vi "Serial_ini.vi"(6 "error in":errorcluster, 7 "Serial path":path, 8 "Date":string, 9 "Count":i32, 10 "Shift":string, 11 "Enum":enum16{"Write", "Read"}(ring)) -> (0 "error out":errorcluster, 1 "Count":u32, 2 "Shift":string, 3 "Date":string)   [LabVIEW 2017]
uses:
  <vilib>/Utility/config.llb/Write Key (String).vi
  <vilib>/Utility/config.llb/Write Key (I32).vi
  <vilib>/Utility/config.llb/Read Key (String).vi
  <vilib>/Utility/config.llb/Read Key (U32).vi
  <vilib>/Utility/config.llb/NI_LVConfig.lvlib
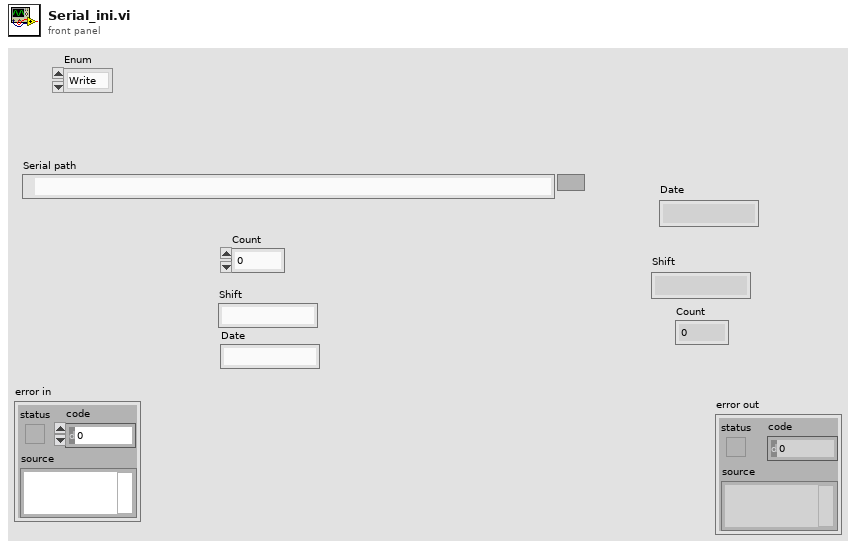
[diagram p1: front panel]
types:
  T1 = typedef "NI_LVConfig.lvlib/Config Data RefNum.ctl" = refnum<k1>
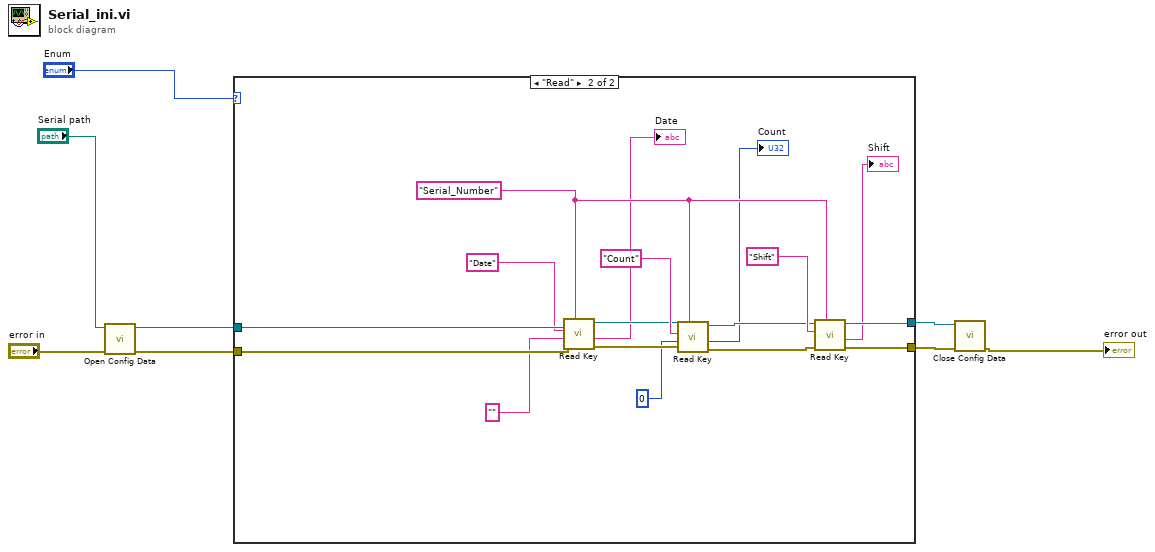
[diagram p0: block diagram]
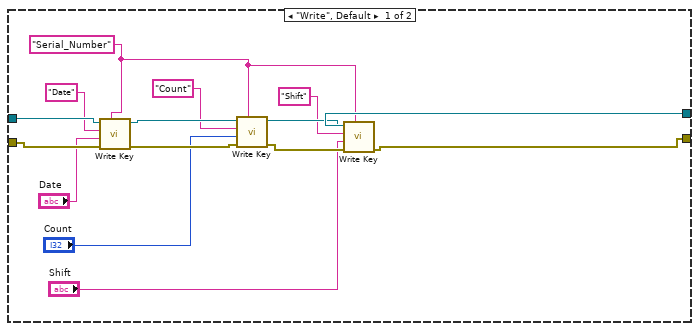
[diagram p2: hidden frame]
diagram:
  n1 = call <vilib>:"Open Config Data.vi"("error in (no error)"="error in", "configuration file path"="Serial path") -> ("error out"=w7:errorcluster, "refnum"=w8:T1)  [unwired: 7 in, 1 out]
  n2 = case shown="\"Read\"" "Enum" {
    tunnel: w7 -> [w23 w40]
    tunnel: w8 -> [w22 w39]
    tunnel: [w19 w31] -> w4
    tunnel: [w18 w29] -> w3
    frame "Write", Default {
      w15 = "Serial_Number" ("name or relative path")
      n3 = call-poly <vilib>:"Write Key.vi"("section"=w15, "error in (no error)"=w23, "value"="Date", "key"="Date" ("name or relative path"), "refnum"=w22) -> ("error out"=w20:errorcluster, "refnum out"=w16:T1)  [unwired: 4 in, 1 out]
      n4 = call-poly <vilib>:"Write Key.vi"("section"=w15, "error in (no error)"=w20, "value"="Count", "key"="Count", "refnum"=w16) -> ("error out"=w21:errorcluster, "refnum out"=w17:T1)  [unwired: 4 in, 1 out]
      n5 = call-poly <vilib>:"Write Key.vi"("section"=w15, "error in (no error)"=w21, "value"="Shift", "key"="Shift", "refnum"=w17) -> ("error out"=w19:errorcluster, "refnum out"=w18:T1)  [unwired: 4 in, 1 out]
    }
    frame "Read" {
      w28 = "Serial_Number" ("name or relative path")
      n6 = call-poly <vilib>:"Read Key.vi"("section"=w28, "error in (no error)"=w40, "default value"="", "key"="Date" ("name or relative path"), "refnum"=w39) -> ("error out"=w36:errorcluster, "value"=→"Date":string, "refnum out"=w37:T1)  [unwired: 3 in, 1 out]
      n7 = call-poly <vilib>:"Read Key.vi"("section"=w28, "error in (no error)"=w36, "default value"=u32 0, "key"="Count", "refnum"=w37) -> ("error out"=w32:errorcluster, "value"=→"Count":u32, "refnum out"=w30:T1)  [unwired: 3 in, 1 out]
      n8 = call-poly <vilib>:"Read Key.vi"("section"=w28, "error in (no error)"=w32, "key"="Shift", "refnum"=w30) -> ("error out"=w31:errorcluster, "value"=→"Shift":string, "refnum out"=w29:T1)  [unwired: 4 in, 1 out]
    }
  }
  n9 = call <vilib>:"Close Config Data.vi"("error in (no error)"=w4, "refnum"=w3) -> ("error out"=→"error out":errorcluster)  [unwired: 8 in, 1 out]
